vi "Verify Arduino Libraries.vi"(8 "Error In":errorcluster, 10 "Arduino Base Path":path=path "C:/Program Files (x86)/Arduino") -> (0 "Error Out":errorcluster, 2 "Libraries Exst?":bool, 3 "Path to Arduino\\libraries":path)   [LabVIEW 2014, in "LMH-LINX.lvlib"]
uses:
  <vilib>/MakerHub/LINX/LMH-LINX.lvlib
  <vilib>/regexp/Match Regular Expression.xnode
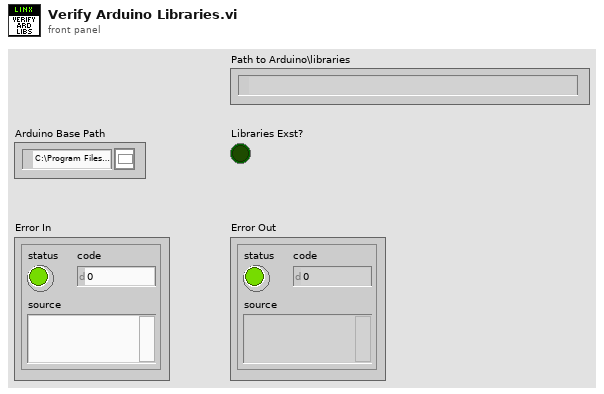
[diagram p1: front panel]
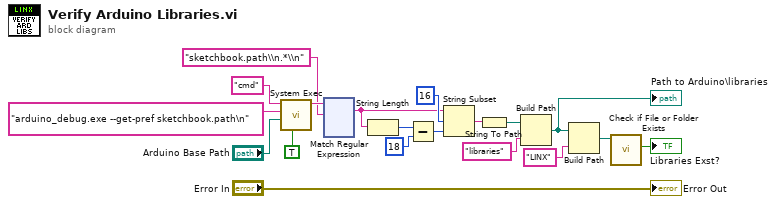
[diagram p0: block diagram]
diagram:
  n1 = call <vilib>:"System Exec.vi"("run minimized? (F)"=TRUE, "working directory"="Arduino Base Path", "standard input"="arduino_debug.exe --get-pref sketchbook.path\n", "command line"="cmd") -> ("standard output"=w15:string)  [unwired: 4 in, 3 out]
  n2 = xnode "Match Regular Expression"("input string"=w15, "regular expression"="sketchbook.path\\n.*\\n") -> ("whole match"=w9:string)  [unwired: 4 in, 4 out]
  n3 = String Length(string=w9) -> (length=w8:i32)
  n4 = Subtract(x=w8, y=18) -> (x-y=w6:i32)
  n5 = String Subset(string=w9, offset (0)=16, length (rest)=w6) -> (substring=w12:string)
  n6 = String To Path(string=w12) -> (path=w11:path)
  n7 = Build Path(base path=w11, name or relative path="libraries") -> (appended path=w5:path)
  "Path to Arduino\\libraries" <- w5
  n8 = Build Path(base path=w5, name or relative path="LINX") -> (appended path=w3:path)
  n9 = call <vilib>:"Check if File or Folder Exists.vi"("path"=w3) -> ("file or folder exists?"=→"Libraries Exst?":bool)  [unwired: 8 in, 2 out]
  "Error Out" <- "Error In"
